vi "Generator blok danych.vi"(6 "Liczba cykli":dbl, 7 "Faza":dbl, 9 "Amplituda":dbl, 10 "Liczba probek":i32, 11 "Sygnal":T1(ring)) -> (3 "Wyjscie":dbl[](array[numeric]))   [LabVIEW 2019]
uses:
  <vilib>/Analysis/NI_AALBase.lvlib
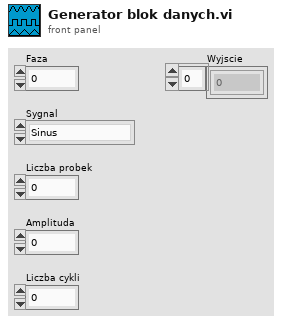
[diagram p1: front panel]
types:
  T1 = enum16{"Sinus", "Prostokąt", "Piła", "Trójkąt", "Rozkład losowy", "Rozkład normalny"}
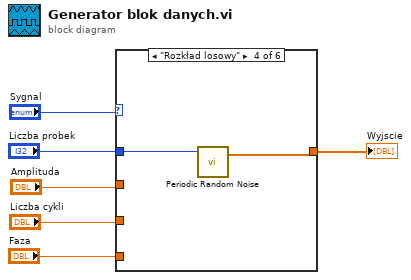
[diagram p0: block diagram]
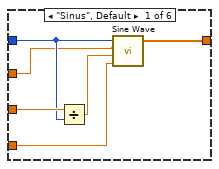
[diagram p2: hidden frame]
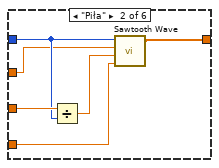
[diagram p3: hidden frame]
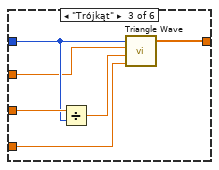
[diagram p4: hidden frame]
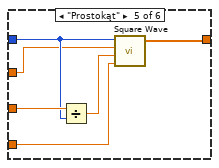
[diagram p5: hidden frame]
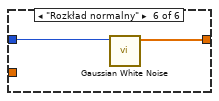
[diagram p6: hidden frame]
diagram:
  n1 = case shown="\"Rozkład losowy\"" "Sygnal" {
    tunnel: "Liczba probek" -> [w11 w16 w22 w26 w30 w34]
    tunnel: "Amplituda" -> [w10 w14 w19 _ w28 _]
    tunnel: "Liczba cykli" -> [w12 w17 w23 _ w31 _]
    tunnel: "Faza" -> [w8 w13 w20 _ w27 _]
    tunnel: [w7 w18 w24 w25 w32 w33] -> w6
    frame "Sinus", Default {
      n2 = Divide(x=w12, y=w11) -> (x/y=w9:dbl)
      n3 = call <vilib>:"Sine Wave.vi"("samples"=w11, "amplitude"=w10, "frequency"=w9, "phase in"=w8) -> ("sine wave"=w7:dbl[])  [unwired: 1 in, 2 out]
    }
    frame "Piła" {
      n4 = Divide(x=w17, y=w16) -> (x/y=w15:dbl)
      n5 = call <vilib>:"Sawtooth Wave.vi"("samples"=w16, "amplitude"=w14, "frequency"=w15, "phase in"=w13) -> ("sawtooth wave"=w18:dbl[])  [unwired: 1 in, 2 out]
    }
    frame "Trójkąt" {
      n6 = Divide(x=w23, y=w22) -> (x/y=w21:dbl)
      n7 = call <vilib>:"Triangle Wave.vi"("samples"=w22, "amplitude"=w19, "frequency"=w21, "phase in"=w20) -> ("triangle wave"=w24:dbl[])  [unwired: 1 in, 2 out]
    }
    frame "Rozkład losowy" {
      n8 = call <vilib>:"Periodic Random Noise.vi"("samples"=w26) -> ("periodic random noise"=w25:dbl[])  [unwired: 2 in, 1 out]
    }
    frame "Prostokąt" {
      n9 = Divide(x=w31, y=w30) -> (x/y=w29:dbl)
      n10 = call <vilib>:"Square Wave.vi"("samples"=w30, "amplitude"=w28, "frequency"=w29, "phase in"=w27) -> ("square wave"=w32:dbl[])  [unwired: 2 in, 2 out]
    }
    frame "Rozkład normalny" {
      n11 = call <vilib>:"Gaussian White Noise.vi"("samples"=w34) -> ("Gaussian noise pattern"=w33:dbl[])  [unwired: 9 in, 1 out]
    }
  }
  "Wyjscie" <- w6
